vi "Test Close Logging.vi"(8 "error in":errorcluster) -> (0 "error out":errorcluster)   [LabVIEW 2016, in "UT_Helper.lvlib"]
doc: "Test if there is no error after an existent Logger was closed.\nTest if there is an error after the close was called again."
uses:
  UT_Helper.lvlib
  Source/HSE-Logger/Handler/Handler.lvclass
  Source/HSE-Logger/hse-logger.lvlib
  <vilib>/addons/_JKI Toolkits/Caraya/classes/Test/Test.lvclass
  <vilib>/addons/_JKI Toolkits/Caraya/classes/Assert/Assert.lvclass
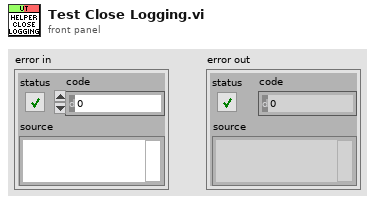
[diagram p1: front panel]
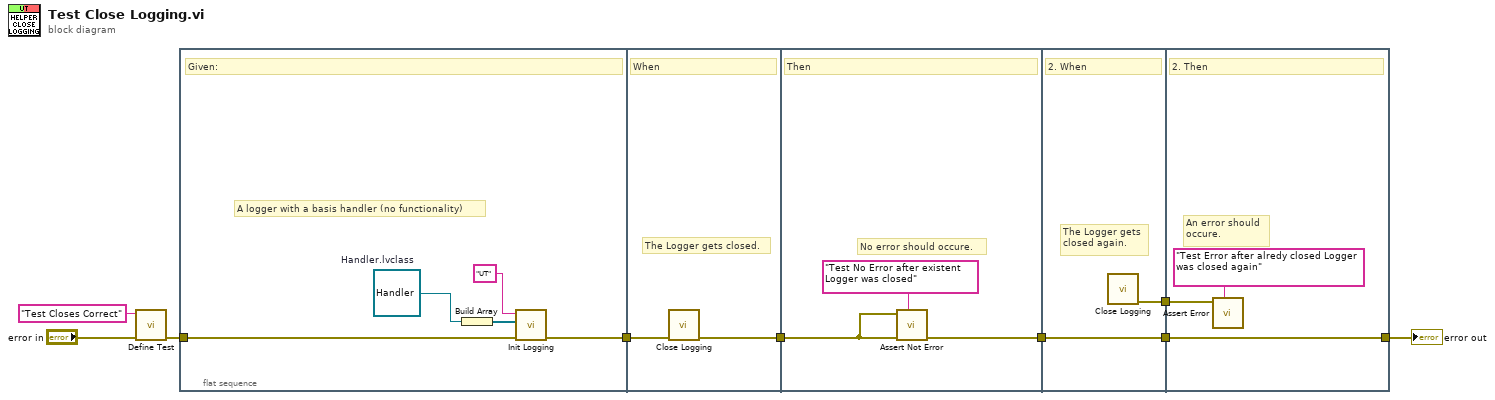
[diagram p0: block diagram]
diagram:
  n1 = call <vilib>:"Define Test.vi"("error in (no error)"="error in", "Label (VI Title)"="Test Closes Correct") -> ("error out"=w5:errorcluster)  [unwired: 8 in, 1 out]
  n2 = flat-sequence {
    tunnel: w5 -> [w14]
    tunnel: [w13] -> w9
    tunnel: w9 -> [w16]
    tunnel: [w15] -> w8
    tunnel: w8 -> [w18]
    tunnel: [w19] -> w4
    tunnel: w4 -> [w20]
    tunnel: [w21] -> w3
    tunnel: [w20] -> w2
    tunnel: [w23] -> w7
    tunnel: w3 -> [w24]
    tunnel: w2 -> [w23]
    frame #0 {
      w11 = refnum<class "Handler.lvclass"> refnum  # Handler.lvclass
      # "A logger with a basis handler (no functionality)"
      # "Given:"
      n3 = Build Array(w11) -> (w10:refnum<class "Handler.lvclass">[])
      n4 = call "Init Logging.vi"("error in"=w14, "Handlers"=w10, "Name"="UT") -> ("error out"=w13:errorcluster)  [unwired: 8 in]
    }
    frame #1 {
      # "The Logger gets closed."
      # "When"
      n5 = call "Close Logging.vi"("error in"=w16) -> ("error out"=w15:errorcluster)  [unwired: 10 in]
    }
    frame #2 {
      # "No error should occure."
      # "Then"
      n6 = call <vilib>:"Assert Not Error.vi"("Label"="Test No Error after existent Logger was closed", "error in (no error)"=w18, "Not Error?"=w18) -> ("error out"=w19:errorcluster)  [unwired: 7 in, 1 out]
    }
    frame #3 {
      # "The Logger gets\nclosed again."
      # "2. When"
      n7 = call "Close Logging.vi"() -> ("error out"=w21:errorcluster)  [unwired: 11 in]
    }
    frame #4 {
      # "An error should\noccure."
      # "2. Then"
      n8 = call <vilib>:"Assert Error.vi"("Label"="Test Error after alredy closed Logger was closed again", "Error?"=w24) -> ()  [unwired: 8 in, 2 out]
    }
  }
  "error out" <- w7
